vi "Tracker_TTL_swap_speed_test.vi"() -> ()   [LabVIEW 2018]
panel:
  in  "milliseconds to wait":u32
  in  "Stop":bool
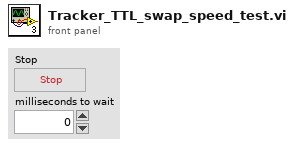
[diagram p1: front panel]
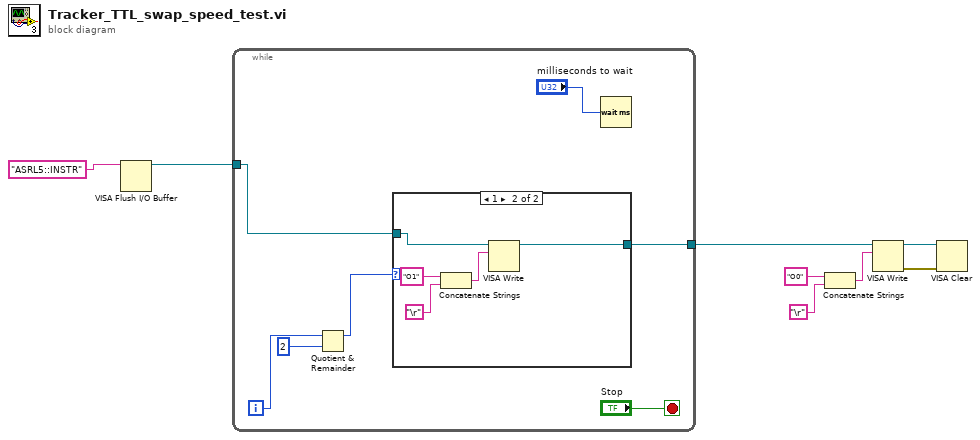
[diagram p0: block diagram]
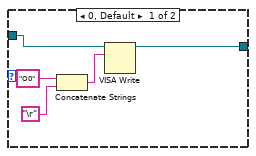
[diagram p2: hidden frame]
diagram:
  n1 = VISA Flush I/O Buffer(VISA resource name="ASRL5::INSTR" ("Resource")) -> (VISA resource name out=w7:refnum<visa-resource-name>)  [unwired: 2 in, 1 out]
  n2 = while {
    tunnel: w7 -> [w10]
    tunnel: [w9] -> w3
    i -> [w13]
    stop <- "Stop" stop-if-true
    n3 = Quotient & Remainder(x=w13, y=2) -> (x-y*floor(x/y)=w11:i32)  [unwired: 1 out]
    n4 = case shown="1" w11 {
      tunnel: w10 -> [w20 w25]
      tunnel: [w16 w21] -> w9
      frame 0, Default {
        n5 = Concatenate Strings("O0" ("string"), "\r") -> (w17:string)
        n6 = VISA Write(VISA resource name=w20, write buffer=w17) -> (VISA resource name out=w16:refnum<visa-resource-name>)  [unwired: 1 in, 2 out]
      }
      frame 1 {
        n7 = Concatenate Strings("O1" ("string"), "\r") -> (w22:string)
        n8 = VISA Write(VISA resource name=w25, write buffer=w22) -> (VISA resource name out=w21:refnum<visa-resource-name>)  [unwired: 1 in, 2 out]
      }
    }
    n9 = Wait (ms)(milliseconds to wait="milliseconds to wait") -> ()  [unwired: 1 out]
  }
  n10 = Concatenate Strings("O0" ("string"), "\r") -> (w6:string)
  n11 = VISA Write(VISA resource name=w3, write buffer=w6) -> (VISA resource name out=w2:refnum<visa-resource-name>, error out=w1:errorcluster)  [unwired: 1 in, 1 out]
  n12 = VISA Clear(VISA resource name=w2, error in (no error)=w1) -> ()  [unwired: 2 out]
